vi "rosearray.vi"(4 "Iterations":u32=1000 step=100, 5 "number of periods":dbl=1.0 format="%.2f", 6 "c":dbl format="%.2f", 7 "b":dbl=1000.0 step=1.0 format="%.2f", 8 "a":dbl=4.0 step=1.0 format="%.2f") -> (1 "Y Array":dbl[](array[numeric]), 2 "X Array":dbl[](array[numeric]), 3 "Array":dbl[](array[numeric]) format="%.2f")   [LabVIEW 2014]
panel:
  out "XY Graph":cluster{dbl, dbl}[](graph)
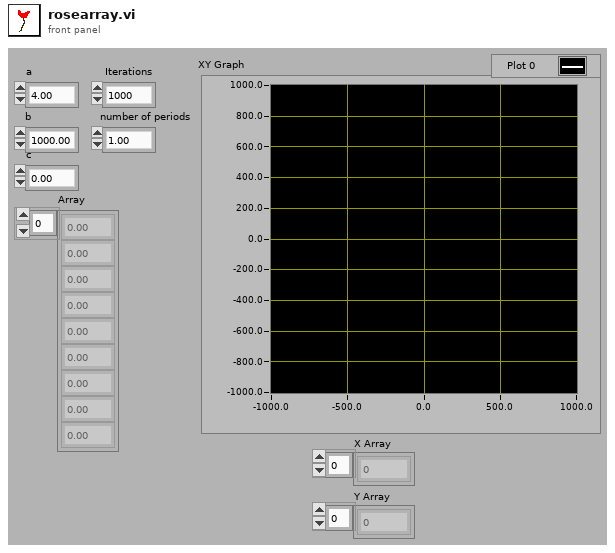
[diagram p1: front panel]
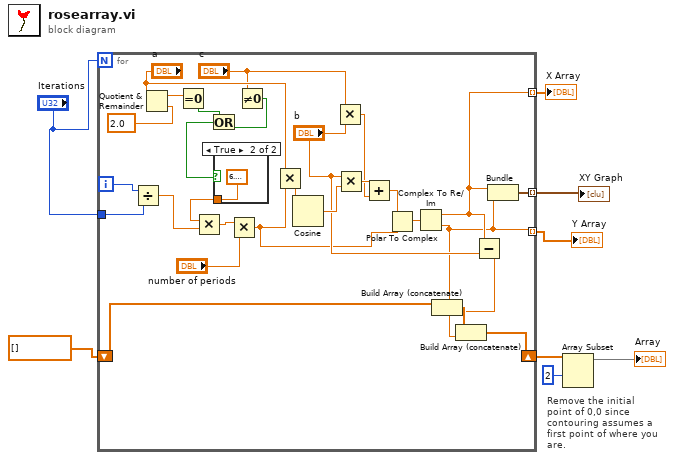
[diagram p0: block diagram]
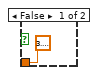
[diagram p2: hidden frame]
diagram:
  # "Remove the initial point of 0,0 since contouring assumes a first point of where you are."
  n1 = for {
    N: "Iterations" -> [_]
    tunnel: "Iterations" -> [w35]
    shift-right: [w28] -> w4
    shift-left: dbl[] [] -> [w30]
    tunnel: [w14] -> w7 mode=indexing
    tunnel: [w10] -> w2 mode=indexing
    tunnel: [w9] -> w1 mode=indexing
    i -> [w36]
    n2 = Divide(x=w36, y=w35) -> (x/y=w23:dbl)
    n3 = Quotient & Remainder(x="a", y=2.0) -> (x-y*floor(x/y)=w25:dbl)  [unwired: 1 out]
    n4 = Equal To 0?(x=w25) -> (x = 0?=w24:bool)
    n5 = Not Equal To 0?(x="c") -> (x != 0?=w18:bool)
    n6 = Or(x=w24, y=w18) -> (x .or. y?=w20:bool)
    n7 = case shown="True" w20 {
      tunnel: [3.141592653589793 6.283185307179586] -> w22
      frame False {
      }
      frame True {
      }
    }
    n8 = Multiply(x=w22, y=w23) -> (x*y=w31:dbl)
    n9 = Multiply(x=w31, y="number of periods") -> (x*y=w11:dbl)
    n10 = Multiply(x="a", y=w11) -> (x*y=w32:dbl)
    n11 = Cosine(x=w32) -> (cos(x)=w34:dbl)
    n12 = Multiply(x="c", y="b") -> (x*y=w21:dbl)
    n13 = Multiply(x="b", y=w34) -> (x*y=w33:dbl)
    n14 = Add(x=w33, y=w21) -> (x+y=w12:dbl)
    n15 = Polar To Complex(1:w11, 2:w12) -> (0:w13:cdb)
    n16 = Complex To Re/Im(x + iy=w13) -> (x=w10:dbl, y=w9:dbl)
    n17 = Subtract(x=w10, y="b") -> (x-y=w16:dbl)
    n18 = Build Array (concatenate)(w30, w16) -> (w29:dbl[])
    n19 = Build Array (concatenate)(w29, w9) -> (w28:dbl[])
    n20 = Bundle(w10, w9) -> (w14:cluster{dbl, dbl})  [unwired: 1 in]
  }
  "XY Graph" <- w7
  "X Array" <- w2
  "Y Array" <- w1
  n21 = Array Subset(array=w4, index=2 ("Array Index")) -> (→"Array":dbl[])  [unwired: 1 in]
